vi "VIPBuild.vi"() -> ()   [LabVIEW 2011, in "G CLI VIP.lvlib"]
uses:
  G CLI VIP.lvlib
  <vilib>/Wiresmith Technology/G CLI/Argument Parser/Option Class/Option Configuration.ctl
  <vilib>/Wiresmith Technology/G CLI/Argument Parser/Option Class/Argument Type.ctl
  <vilib>/Wiresmith Technology/G CLI/CLI Class/CLI.lvclass
  <vilib>/Wiresmith Technology/G CLI/Argument Parser/Option Set Class/Option Set.lvclass
  <vilib>/Wiresmith Technology/G CLI/Argument Parser/Option Class/Option.lvclass
  <vilib>/JKI/VIPM API/VIPM API_vipm_api.lvlib
panel:
  out "error out":errorcluster
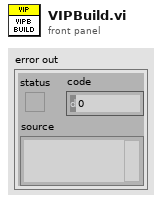
[diagram p1: front panel]
types:
  T1 = typedef "Option Parser.lvlib/Option.lvclass/Option Configuration.ctl" = cluster{"Option Type":T2, "Option Labels":string[], "Key":string, "Description":string, "Required":bool, "Default Value":string}
  T2 = typedef "Option Parser.lvlib/Option.lvclass/Argument Type.ctl" = enum16{"flag", "value"}
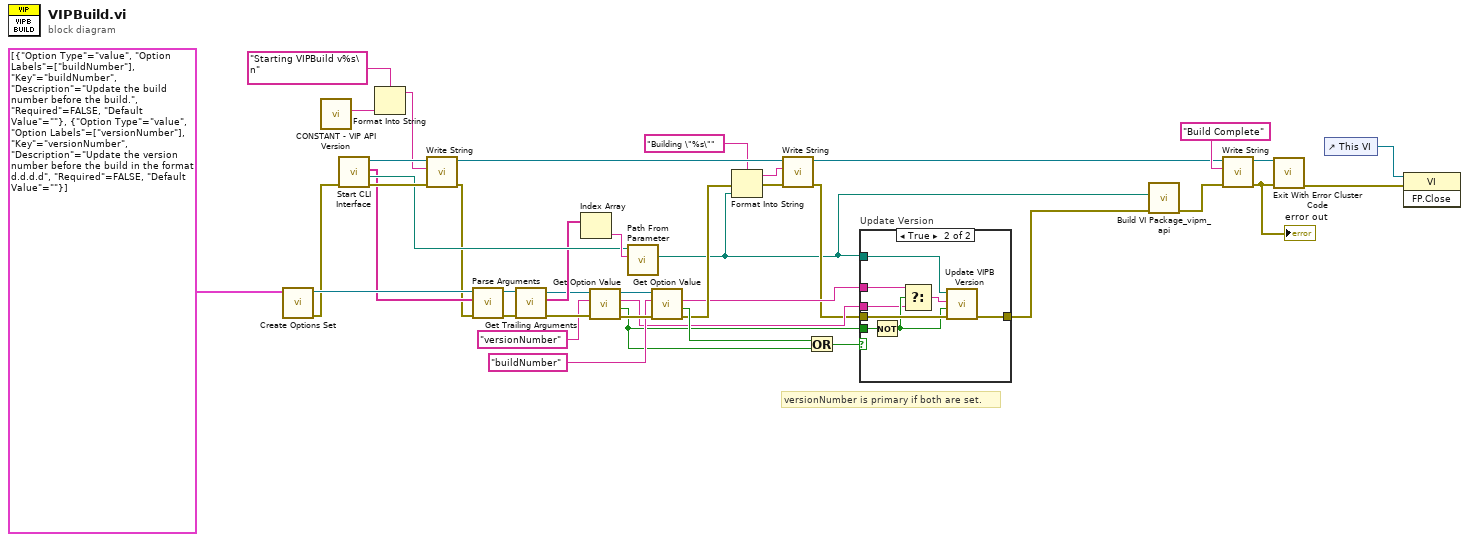
[diagram p0: block diagram]
diagram:
  # "versionNumber is primary if both are set."
  n1 = call <vilib>:"Create Options Set.vi"("Options"=T1[] [{"Option Type"=enum."value", "Option Labels"=["buildNumber"], "Key"="buildNumber", "Description"="Update the build number before the build.", "Required"=FALSE, "Default Value"=""}, {"Option Type"=enum."value", "Option Labels"=["versionNumber"], "Key"="versionNumber", "Description"="Update the version number before the build in the format d.d.d.d", "Required"=FALSE, "Default Value"=""}]) -> ("error out"=w22:errorcluster, "Option Set out"=w29:refnum<class "Option Set.lvclass">)  [unwired: 9 in]
  n2 = call "CONSTANT - VIP API Version.vi"() -> ("Version"=w38:string)  [unwired: 11 in]
  n3 = call <vilib>:"Start CLI Interface.vi"("error in (no error)"=w22) -> ("error out"=w40:errorcluster, "Working Directory"=w34:path, "Custom Parameters"=w28:string[], "CLI out"=w41:refnum<class "CLI.lvclass">)  [unwired: 7 in]
  n4 = Format Into String(format string="Starting VIPBuild v%s\n", w38) -> (resulting string=w37:string)  [unwired: 2 in, 1 out]
  n5 = call <vilib>:"Write String.vi"("error in (no error)"=w40, "Text to Write"=w37, "CLI in"=w41) -> ("error out"=w21:errorcluster, "CLI out"=w6:refnum<class "CLI.lvclass">)  [unwired: 7 in]
  n6 = call <vilib>:"Parse Arguments.vi"("error in (no error)"=w21, "Arguments"=w28, "Option Set in"=w29) -> ("error out"=w27:errorcluster, "Option Set out"=w26:refnum<class "Option Set.lvclass">)  [unwired: 5 in, 2 out]
  n7 = call <vilib>:"Get Trailing Arguments.vi"("error in (no error)"=w27, "Option Set in"=w26) -> ("error out"=w23:errorcluster, "Arguments"=w25:string[], "Option Set out"=w24:refnum<class "Option Set.lvclass">)  [unwired: 7 in]
  n8 = Index Array(array=w25) -> (element=w35:string)  [unwired: 1 in]
  n9 = call <vilib>:"Get Option Value.vi"("error in (no error)"=w23, "Option Key"="versionNumber", "Option Set in"=w24) -> ("error out"=w19:errorcluster, "Set"=w12:bool, "Value"=w10:string, "Option Set out"=w18:refnum<class "Option Set.lvclass">)  [unwired: 5 in]
  n10 = call <vilib>:"Path From Parameter.vi"("Path Parameter"=w35, "Working Directory"=w34) -> ("Full Path"=w1:path)  [unwired: 9 in]
  n11 = call <vilib>:"Get Option Value.vi"("error in (no error)"=w19, "Option Key"="buildNumber", "Option Set in"=w18) -> ("error out"=w14:errorcluster, "Set"=w16:bool, "Value"=w11:string)  [unwired: 5 in, 1 out]
  n12 = Format Into String(format string="Building \"%s\"", error in=w14, w1) -> (resulting string=w3:string, error out=w4:errorcluster)  [unwired: 1 in]
  n13 = call <vilib>:"Write String.vi"("error in (no error)"=w4, "Text to Write"=w3, "CLI in"=w6) -> ("error out"=w7:errorcluster, "CLI out"=w5:refnum<class "CLI.lvclass">)  [unwired: 7 in]
  n14 = Or(x=w16, y=w12) -> (x .or. y?=w13:bool)
  n15 = case "Update Version" shown="True" w13 {
    tunnel: [w42 w50] -> w15
    tunnel: w7 -> [w42 w49]
    tunnel: w1 -> [_ w48]
    tunnel: w12 -> [_ w47]
    tunnel: w11 -> [_ w45]
    tunnel: w10 -> [_ w44]
    frame False {
    }
    frame True {
      n16 = Not(x=w47) -> (.not. x?=w46:bool)
      n17 = Select(t=w45, s=w46, f=w44) -> (s? t:f=w43:string)
      n18 = call "Update VIPB Version.vi"("error in (no error)"=w49, "Build Only"=w46, "New Version"=w43, "Full Path"=w48) -> ("error out"=w50:errorcluster)  [unwired: 7 in]
    }
  }
  n19 = call <vilib>:"Build VI Package_vipm_api.vi"("error in (no error)"=w15, "Path to VIPB File"=w1) -> ("error out"=w36:errorcluster)  [unwired: 8 in, 1 out]
  n20 = call <vilib>:"Write String.vi"("error in (no error)"=w36, "Text to Write"="Build Complete", "CLI in"=w5) -> ("error out"=w33:errorcluster, "CLI out"=w32:refnum<class "CLI.lvclass">)  [unwired: 7 in]
  "error out" <- w33
  n21 = call <vilib>:"Exit With Error Cluster Code.vi"("error in (no error)"=w33, "CLI in"=w32) -> ("error out"=w8:errorcluster)  [unwired: 9 in]
  n22 = control-ref of="This VI"() -> (w9:refnum<vi>)
  n23 = invoke class="VI" method="FP.Close"(reference=w9, error in=w8) -> ()  [unwired: 1 in, 3 out]
